vi "Display and Log reading file errror.vi"(8 "Error In":errorcluster, 11 "Action":string="Loadplus Device Setting config") -> (0 "error out":errorcluster)   [LabVIEW 2019]
uses:
  3e670435-1843-48d2-b087-6f430162fdf0.vi
  Appplicaiton Enviroment/SubVI/Get Development Mode.vi
  User Interface Logger/SubVI/Data Types/Log Integer.vi
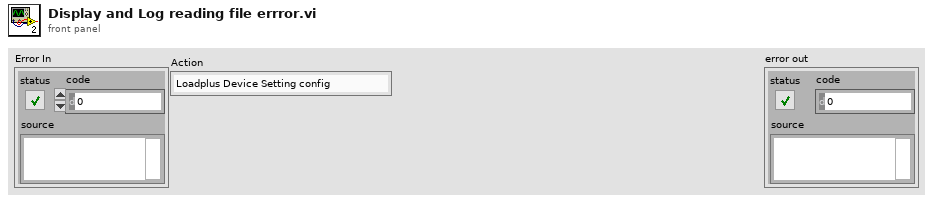
[diagram p1: front panel]
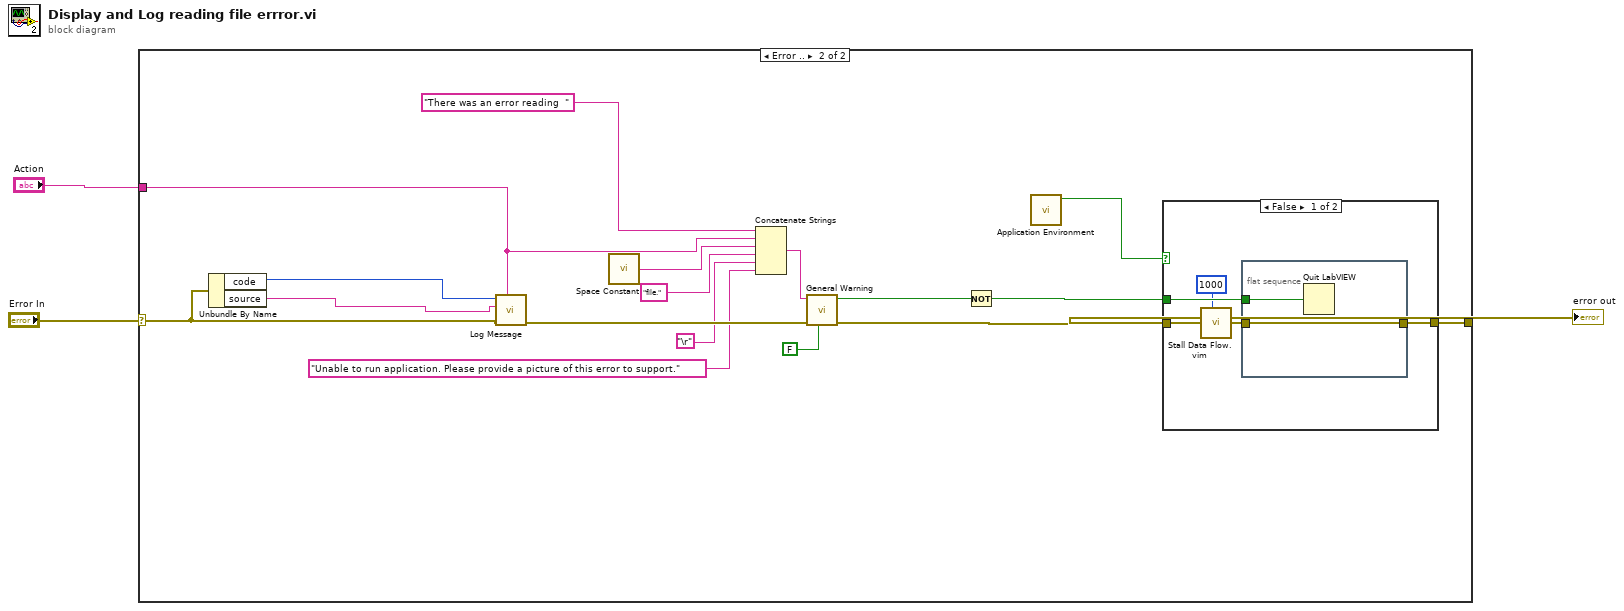
[diagram p0: block diagram]
diagram:
  n1 = case shown="Error .." "Error In" {
    selector: "Error In" -> [w4 w19]
    tunnel: [w4 w10] -> w2
    tunnel: "Action" -> [_ w14]
    frame No Error {
    }
    frame Error {
      n2 = Unbundle By Name(w19) -> ("code"=w21:i32, "source"=w20:string)
      n3 = call-poly "Log Message.vi"("Action"=w14, "error in (no error)"=w19, "Data Field Descriptor"=w20, "number"=w21) -> ("error out"=w18:errorcluster)  [unwired: 7 in]
      n4 = call <vilib>:"Space Constant.vi"() -> ("String"=w12:string)
      n5 = Concatenate Strings("There was an error reading  " ("string"), w14, w12, "file." ("string"), "\r", "Unable to run application. Please provide a picture of this error to support." ("string")) -> (w16:string)
      n6 = call "General Warning.vi"("Show Cancel Button"=FALSE, "error in (no error)"=w18, "WarningMessage"=w16) -> ("error out"=w11:errorcluster, "Cancelled?"=w9:bool)  [unwired: 7 in]
      n7 = Not(x=w9) -> (.not. x?=w8:bool)
      n8 = call-poly "Application Environment.vi"() -> ("Development"=w7:bool)  [unwired: 10 in, 1 out]
      n9 = case shown="False" w7 {
        tunnel: w11 -> [w26 w29]
        tunnel: [w25 w29] -> w10
        tunnel: w8 -> [w24 _]
        frame False {
          n10 = call "Stall Data Flow.vim"("value in"=w26, "milliseconds to wait"=u32 1000) -> ("value out"=w23:errorcluster)  [unwired: 1 out]
          n11 = flat-sequence {
            tunnel: w24 -> [w28]
            tunnel: w23 -> [w27]
            tunnel: [w27] -> w25
            frame #0 {
              n12 = Quit LabVIEW(quit? (T)=w28) -> ()
            }
          }
        }
        frame True {
        }
      }
    }
  }
  "error out" <- w2
